vi "Global 1.vi"() -> ()   [LabVIEW 2020]
panel:
  in  "Numeric":i32
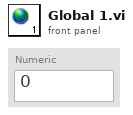
[diagram p1: front panel]
diagram:
